vi "RichToFlatcrio_dashboard_ShutdownResponse.vi"(5 "OutputClusterType":T1, 11 "InputCluster":T2) -> (3 "OutputCluster":T1)   [LabVIEW 2026, in "WebPageInterface_client.lvlib"]
uses:
  WebPageInterface_client.lvlib
  crio_dashboard_ShutdownResponse_Flat.ctl
  crio_dashboard_ShutdownResponse.ctl
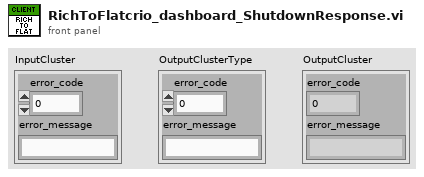
[diagram p1: front panel]
types:
  T1 = typedef "WebPageInterface_client.lvlib/crio_dashboard_ShutdownResponse_Flat.ctl" = cluster{"error_code":i32, "error_message":string}
  T2 = typedef "WebPageInterface_client.lvlib/crio_dashboard_ShutdownResponse.ctl" = cluster{"error_code":i32, "error_message":string}
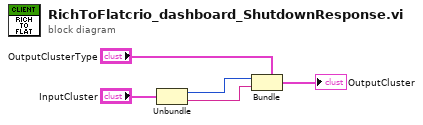
[diagram p0: block diagram]
diagram:
  n1 = Unbundle "Unbundle"("InputCluster") -> ("error_code"=w2:i32, "error_message"=w1:string)
  n2 = Bundle "Bundle"(cluster="OutputClusterType", "error_code"=w2, "error_message"=w1) -> (→"OutputCluster":T1)
